vi "Get Owning Pane of Control.vi"(8 "error in (no error)":errorcluster, 11 "Ctl Refnum":refnum<vi>) -> (0 "error out":errorcluster, 2 "Owning Pane":refnum<vi>, 3 "dup Ctl Refnum":refnum<vi>)   [LabVIEW 2013]
uses:
  <vilib>/Utility/traverseref.llb/TRef TravTarget.ctl
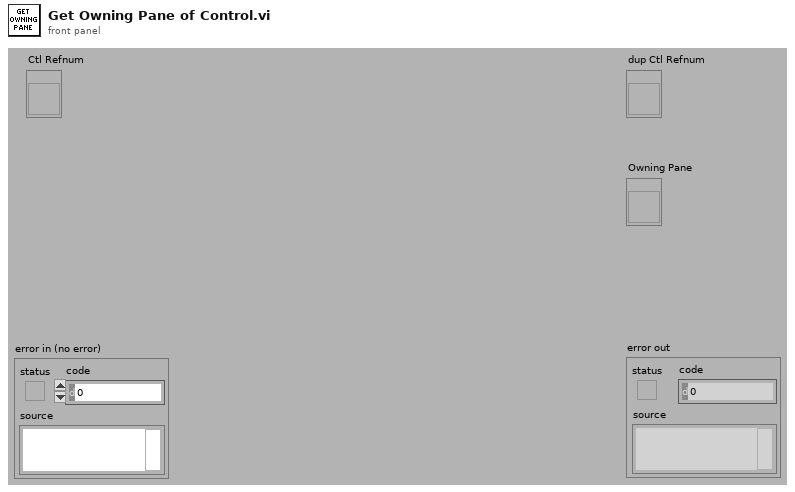
[diagram p1: front panel]
types:
  T1 = typedef "TRef TravTarget.ctl" = enum16{"FP", "BD", "Other"}
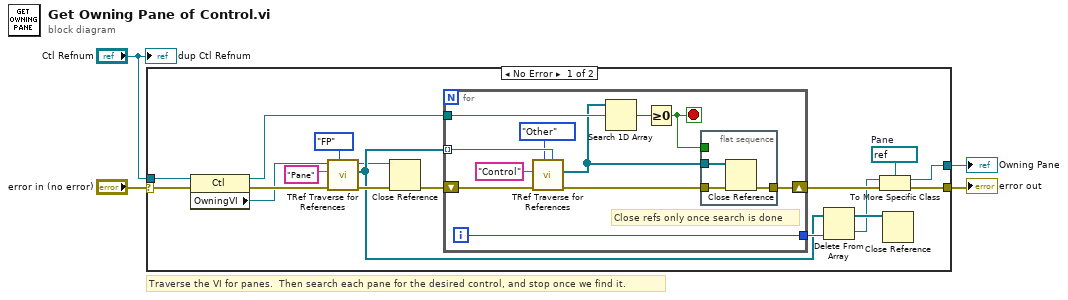
[diagram p0: block diagram]
diagram:
  # "Traverse the VI for panes.  Then search each pane for the desired control, and stop once we find it."
  n1 = case shown="No Error" "error in (no error)" {
    selector: "error in (no error)" -> [w22 w37]
    tunnel: [w11 w37] -> w3
    tunnel: "Ctl Refnum" -> [w21 _]
    tunnel: [w9 _] -> w1
    frame No Error {
      w13 = refnum<vi> refnum  # Pane
      n2 = property class="Ctl"(reference=w21, error in=w22) -> (reference out=w16:refnum<vi>, error out=w20:errorcluster, "OwningVI"=w19:refnum<vi>)
      n3 = call <vilib>:"TRef Traverse for References.vi"("Traverse Target"=TRef_TravTarget."FP", "error in (no error)"=w20, "Class Name"="Pane", "VI Refnum"=w19) -> ("error out"=w8:errorcluster, "References"=w7:refnum<vi>[], "dup VI Refnum"=w5:refnum<vi>)  [unwired: 4 in, 1 out]
      n4 = Close Reference(reference=w5, error in (no error)=w8) -> (error out=w6:errorcluster)
      n5 = for {
        shift-right: [w26] -> w12
        shift-left: w6 -> [w33]
        tunnel: w7 -> [w32] mode=indexing
        tunnel: w16 -> [w29]
        tunnel: [w28] -> w15
        i -> [w28]
        stop <- w23 stop-if-true
        # "Close refs only once search is done"
        n6 = call <vilib>:"TRef Traverse for References.vi"("Other Refnum"=w32, "Traverse Target"=TRef_TravTarget."Other", "error in (no error)"=w33, "Class Name"="Control") -> ("error out"=w25:errorcluster, "References"=w24:refnum<vi>[])  [unwired: 4 in, 2 out]
        n7 = Search 1D Array(1D array=w24, element=w29) -> (index of element=w27:i32)  [unwired: 1 in]
        n8 = Greater Or Equal To 0?(x=w27) -> (x >= 0?=w23:bool)
        n9 = flat-sequence {
          tunnel: [w36] -> w26
          tunnel: w25 -> [w35]
          tunnel: w24 -> [w34]
          tunnel: w23 -> [_]
          frame #0 {
            n10 = Close Reference(reference=w34, error in (no error)=w35) -> (error out=w36:errorcluster)
          }
        }
      }
      n11 = Delete From Array(array=w7, index=w15) -> (deleted portion=w10:refnum<vi>, array with subset deleted=w14:refnum<vi>[])  [unwired: 1 in]
      n12 = To More Specific Class(target class=w13, reference=w10, error in=w12) -> (specific class reference=w9:refnum<vi>, error out=w11:errorcluster)
      n13 = Close Reference(reference=w14) -> ()  [unwired: 1 in, 1 out]
    }
    frame Error {
    }
  }
  "error out" <- w3
  "Owning Pane" <- w1
  "dup Ctl Refnum" <- "Ctl Refnum"
